vi "Array Dedup_2D Str.vi"(6 "정렬?":bool, 8 "error in (no error)":errorcluster caption="에러 입력(에러 없음)", 11 "배열 in":string[][](array[string])) -> (0 "error out":errorcluster caption="에러 출력", 3 "배열 out":string[][](array[string]))   [LabVIEW 2020]
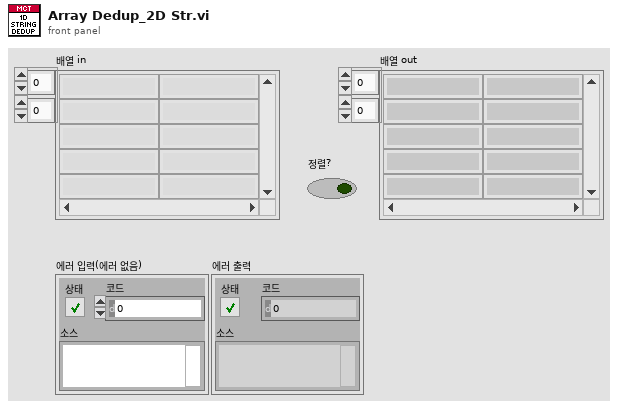
[diagram p1: front panel]
types:
  T1 = cluster{"[0]":string, "[1]":string, "[2]":string, "[3]":string, "[4]":string, "[5]":string, "[6]":string, "[7]":string, "[8]":string}
  T2 = cluster{"[0]":string, "[1]":string, "[2]":string, "[3]":string, "[4]":string, "[5]":string, "[6]":string, "[7]":string, "[8]":string}[]
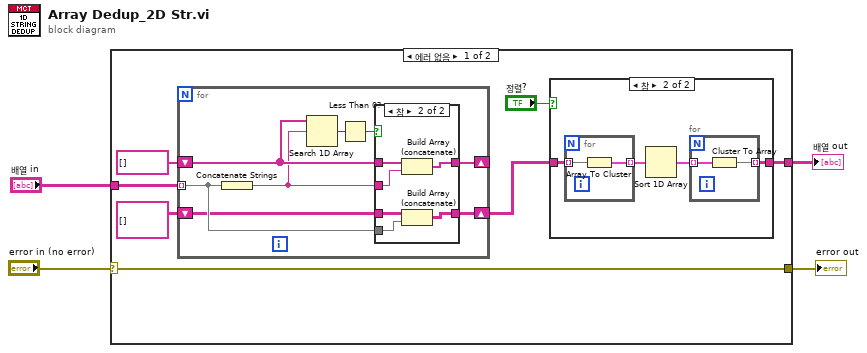
[diagram p0: block diagram]
diagram:
  n1 = case shown="에러 없음" "error in (no error)" {
    selector: "error in (no error)" -> [w10 w37]
    tunnel: "배열 in" -> [w11 w38]
    tunnel: [w6 w38] -> w3
    tunnel: [w10 w37] -> w1
    frame No Error {
      n2 = for {
        tunnel: w11 -> [w23] mode=indexing
        shift-right: [w26] -> _
        shift-left: string[] [] -> [w25]
        shift-right: [w22] -> w7
        shift-left: string[][] [] -> [w21]
        n3 = Concatenate Strings(w23) -> (w24:string)
        n4 = Search 1D Array(1D array=w25, element=w24) -> (index of element=w28:i32)  [unwired: 1 in]
        n5 = Less Than 0?(x=w28) -> (x < 0?=w27:bool)
        n6 = case shown="참" w27 {
          tunnel: [w30 w36] -> w26
          tunnel: w25 -> [w30 w35]
          tunnel: w24 -> [_ w34]
          tunnel: w23 -> [_ w31]
          tunnel: [w29 w33] -> w22
          tunnel: w21 -> [w29 w32]
          frame False {
          }
          frame True {
            n7 = Build Array (concatenate)(w35, w34) -> (w36:string[])
            n8 = Build Array (concatenate)(w32, w31) -> (w33:string[][])
          }
        }
      }
      n9 = case shown="참" "정렬?" {
        tunnel: w7 -> [w12 w16]
        tunnel: [w12 w13] -> w6
        frame False {
        }
        frame True {
          n10 = for {
            tunnel: w16 -> [w20] mode=indexing
            tunnel: [w19] -> w15 mode=indexing
            n11 = Array To Cluster(array=w20) -> (cluster=w19:T1)
          }
          n12 = Sort 1D Array(array=w15) -> (sorted array=w14:T2)
          n13 = for {
            tunnel: w14 -> [w18] mode=indexing
            tunnel: [w17] -> w13 mode=indexing
            n14 = Cluster To Array(cluster=w18) -> (array=w17:string[])
          }
        }
      }
    }
    frame Error {
    }
  }
  "배열 out" <- w3
  "error out" <- w1
